vi "FFT.vi"() -> ()   [LabVIEW 2017]
uses:
  <vilib>/express/express analysis/Spectral/Block/exnSpectralBlock spectral measurements RMS poly.vi
  <vilib>/express/express analysis/Spectral/Block/exnSpectralBlock spectral measurements RMS DDT.vi
  <vilib>/express/express analysis/Spectral/XNode/ExpressSpectralMeasurementsBlockNode.xnode
panel:
  in  "Amplitude":dbl=1.0
  in  "Frequency":dbl=10.1
  out "Spectrum":dynamicdata(graph)
  out "Signal":dynamicdata(graph)
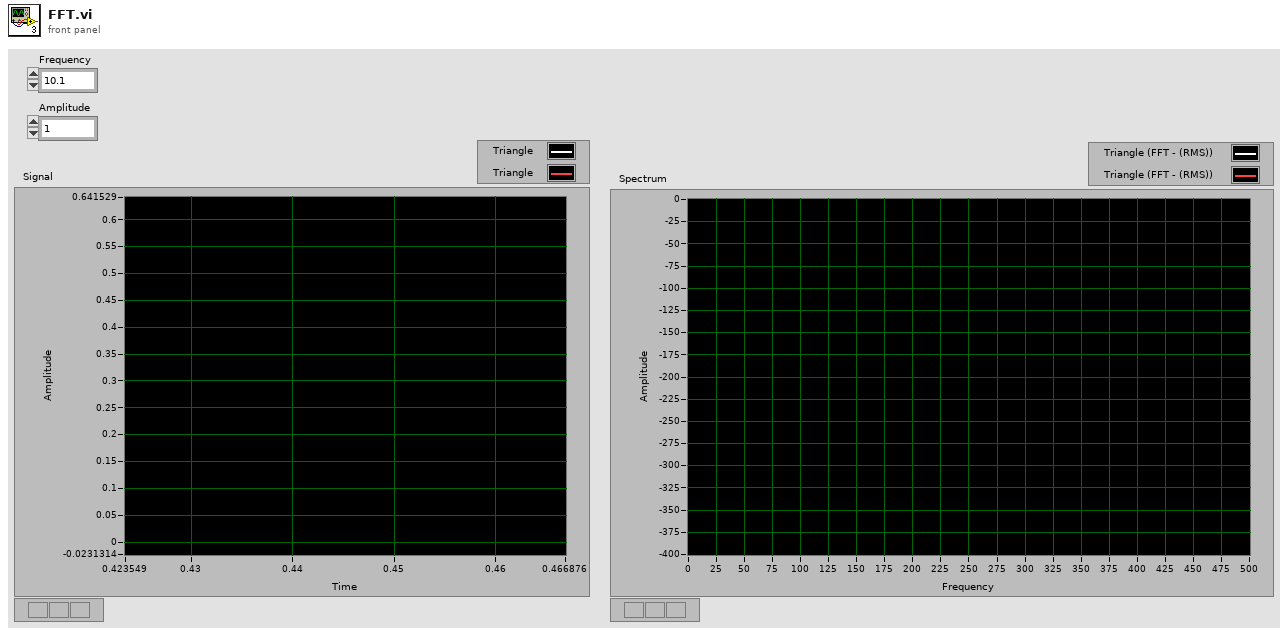
[diagram p1: front panel]
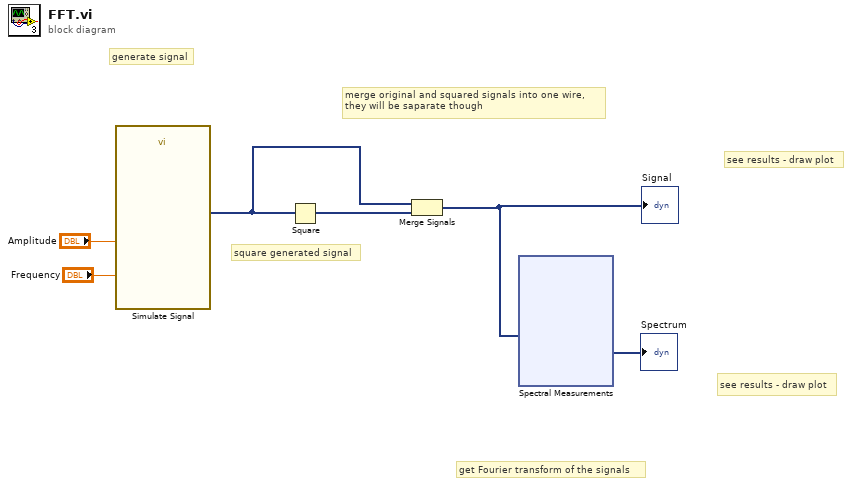
[diagram p0: block diagram]
diagram:
  # "see results - draw plot"
  # "see results - draw plot"
  # "get Fourier transform of the signals"
  # "merge original and squared signals into one wire,\nthey will be saparate though"
  # "square generated signal"
  # "generate signal"
  n1 = call "Simulate Signal"("Frequency"="Frequency", "Amplitude"="Amplitude") -> ("Triangle"=w1:dynamicdata)  [unwired: 12 in, 1 out]
  n2 = Square(x=w1) -> (x^2=w6:dynamicdata)
  n3 = Merge Signals(w1, w6) -> (w4:dynamicdata)
  "Signal" <- w4
  n4 = xnode "Spectral Measurements"("Signals"=w4) -> ("FFT - (RMS)"=→"Spectrum":dynamicdata)  [unwired: 1 in, 2 out]
